vi "Read SDF Path.vi"(8 "error in (no error)":errorcluster, 11 "refnum":T1) -> (0 "error out":errorcluster, 1 "Found?":bool, 2 "Path":path, 3 "refnum out":T1)   [LabVIEW 2016, in "System Mapping Tool.lvlib"]
uses:
  System Mapping Tool.lvlib
  <vilib>/Utility/config.llb/Config Data RefNum.ctl
  <vilib>/Utility/config.llb/Read Key (Path).vi
  <vilib>/Utility/config.llb/NI_LVConfig.lvlib
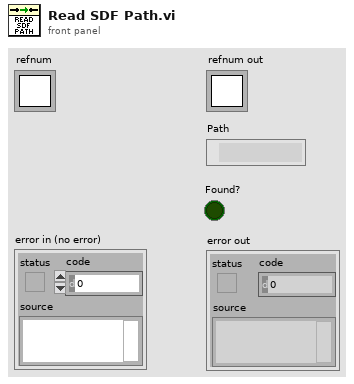
[diagram p1: front panel]
types:
  T1 = typedef "NI_LVConfig.lvlib/Config Data RefNum.ctl" = refnum<k1>
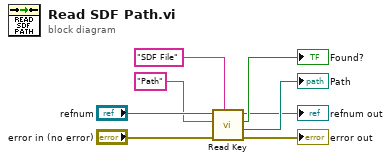
[diagram p0: block diagram]
diagram:
  n1 = call-poly <vilib>:"Read Key.vi"("section"="SDF File", "error in (no error)"="error in (no error)", "key"="Path", "refnum"="refnum") -> ("error out"=→"error out":errorcluster, "value"=→"Path":path, "found?"=→"Found?":bool, "refnum out"=→"refnum out":T1)  [unwired: 4 in]
